vi "initializeCmd.vi"(11 "error in (no error)":errorcluster) -> (4 "cmdSetup":T1, 15 "error out":errorcluster)   [LabVIEW 2017]
uses:
  cmdSetup.ctl
  <vilib>/Utility/config.llb/NI_LVConfig.lvlib
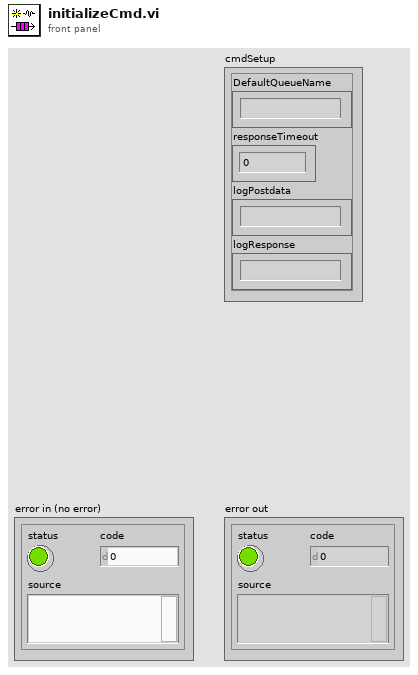
[diagram p1: front panel]
types:
  T1 = typedef "cmdSetup.ctl" = cluster{"DefaultQueueName":string, "responseTimeout":i32, "logPostdata":string, "logResponse":string}
  T2 = typedef "NI_LVConfig.lvlib/Config Data RefNum.ctl" = refnum<k1>
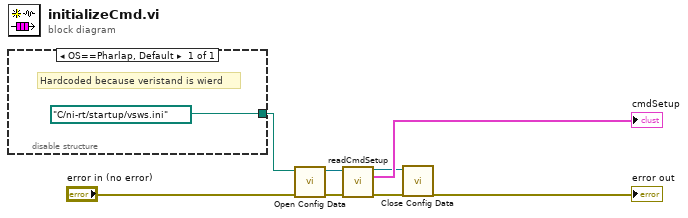
[diagram p0: block diagram]
diagram:
  n1 = disable-structure shown="OS==Pharlap, Default" {
    disable-tunnel: [path "C:/ni-rt/startup/vsws.ini" ("configuration file path")] -> w1
    frame condition #0 (active) {
      # "Hardcoded because veristand is wierd"
    }
  }
  n2 = call <vilib>:"Open Config Data.vi"("error in (no error)"="error in (no error)", "configuration file path"=w1) -> ("error out"=w4:errorcluster, "refnum"=w3:T2)  [unwired: 7 in, 1 out]
  n3 = call "readCmdSetup.vi"("refnum in"=w3, "error in (no error)"=w4) -> ("refnum out"=w5:T2, "cmdSetup"=→"cmdSetup":T1, "error out"=w7:errorcluster)  [unwired: 11 in]
  n4 = call <vilib>:"Close Config Data.vi"("error in (no error)"=w7, "refnum"=w5) -> ("error out"=→"error out":errorcluster)  [unwired: 8 in, 1 out]
